vi "Excel Get Excel Location.vi"(0 "cell's name":string) -> (1 "row":i32, 2 "column":i32)   [LabVIEW 2016, in "NI_ReportGenerationToolkit.lvlib"]
doc: "Returns the row and column indexes of a cell that you identify by Excel syntax."
uses:
  <vilib>/addons/_office/NI_ReportGenerationToolkit.lvlib
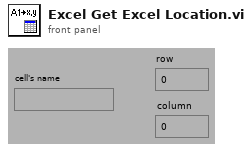
[diagram p1: front panel]
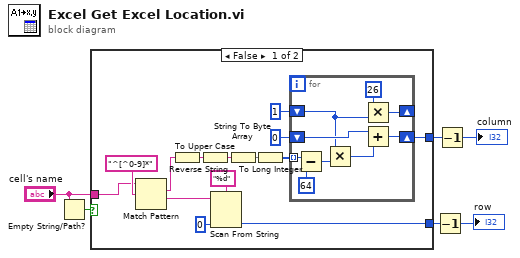
[diagram p0: block diagram]
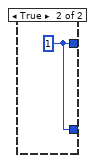
[diagram p2: hidden frame]
diagram:
  n1 = Empty String/Path?(string/path="cell's name") -> (empty?=w3:bool)
  n2 = case shown="False" w3 {
    tunnel: [w13 w30] -> w6
    tunnel: "cell's name" -> [w8 _]
    tunnel: [w7 w30] -> w4
    frame False {
      n3 = Match Pattern(string=w8, regular expression="^[^0-9]*") -> (match substring=w11:string, after substring=w20:string)  [unwired: 1 in, 2 out]
      n4 = To Upper Case(1:w11) -> (0:w14:string)
      n5 = Reverse String(1:w14) -> (0:w16:string)
      n6 = Scan From String(format string="%d" ("Format String"), input string=w20, default 1=0) -> (output 1=w7:i32)  [unwired: 2 in, 3 out]
      n7 = String To Byte Array(string=w16) -> (unsigned byte array=w15:u8[])
      n8 = To Long Integer(number=w15) -> (32bit integer=w9:i32[])
      n9 = for {
        tunnel: w9 -> [w29] mode=indexing
        shift-right: [w25] -> w13
        shift-left: 0 -> [w22]
        shift-right: [w27] -> _
        shift-left: 1 -> [w21]
        n10 = Subtract(x=w29, y=64) -> (x-y=w23:i32)
        n11 = Multiply(x=w21, y=w23) -> (x*y=w24:i32)
        n12 = Multiply(x=26, y=w21) -> (x*y=w27:i32)
        n13 = Add(x=w22, y=w24) -> (x+y=w25:i32)
      }
    }
    frame True {
      w30 = 1
    }
  }
  n14 = Decrement(x=w4) -> (x-1=→"row":i32)
  n15 = Decrement(x=w6) -> (x-1=→"column":i32)
